vi "Current_Calib_Filenames.vi"(3 "Calib Filename":path[](array[path]), 4 "Channel Numbers":string[](array[string]), 5 "Mode":T1) -> (0 "Calib Filename Out":path[](array[path]), 1 "Channel Numbers Out":string[](array[string]))   [LabVIEW 2013]
uses:
  Controls/App_Global.ctl
  File/Setup_Filetype.ctl
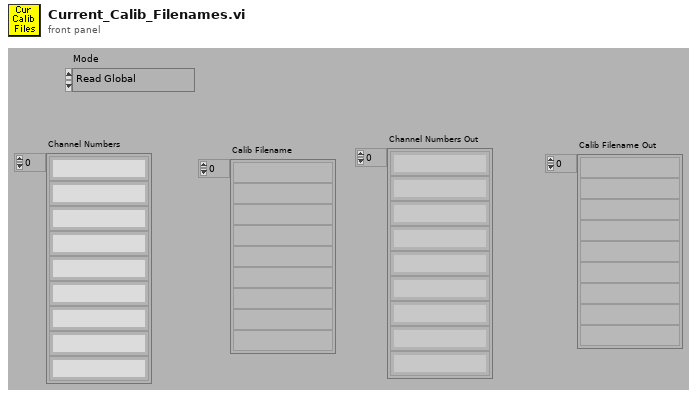
[diagram p1: front panel]
types:
  T1 = typedef "App_Global.ctl" = enum16{"Read Global", "Write to Global", "Initialise Array"}
  T2 = typedef "Setup_Filetype.ctl" = enum16{"Measurement Setups", "Calibration Setups", "General", "Results File Plotter Setups", "Speed Calib Tweaks"}
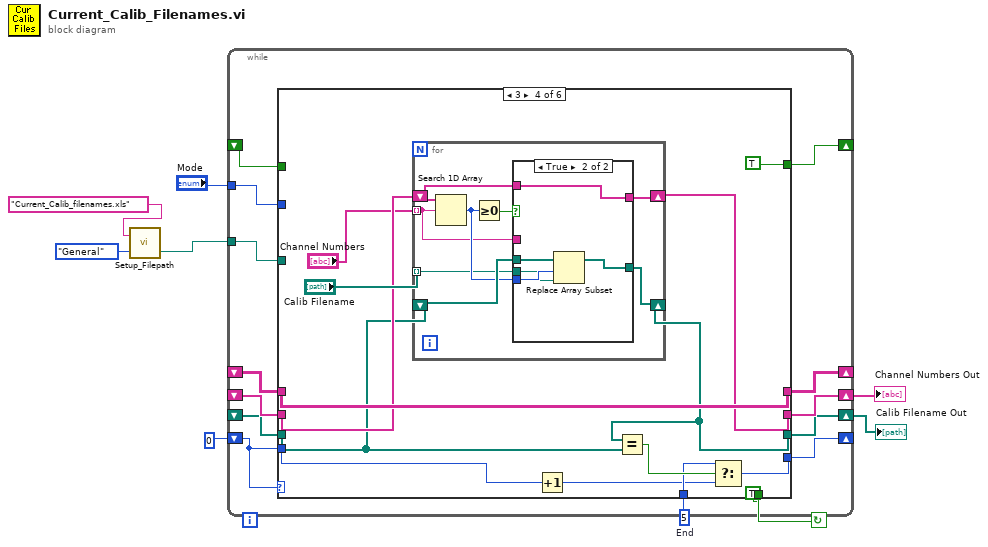
[diagram p0: block diagram]
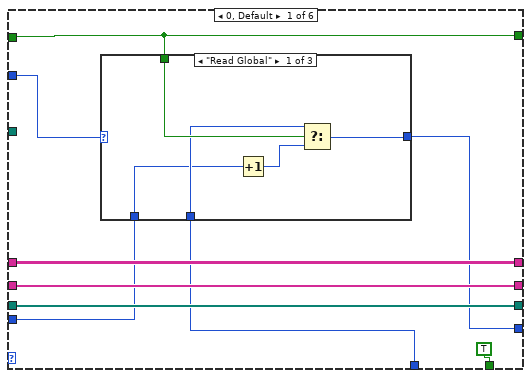
[diagram p2: hidden frame]
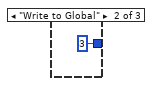
[diagram p3: hidden frame]
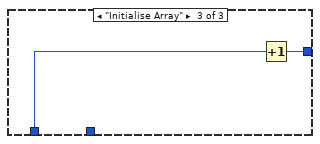
[diagram p4: hidden frame]
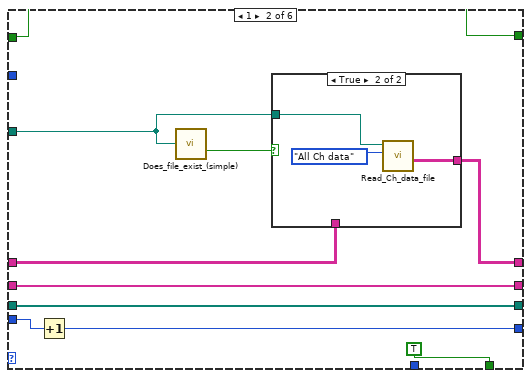
[diagram p5: hidden frame]
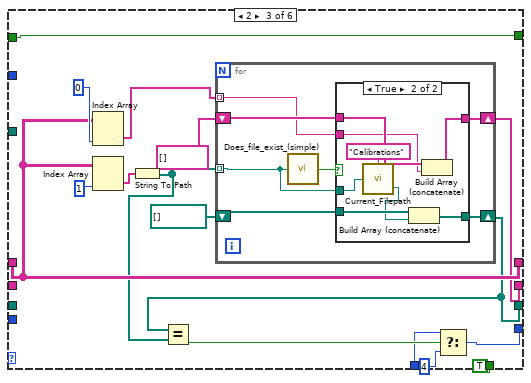
[diagram p7: hidden frame]
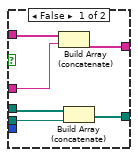
[diagram p9: hidden frame]
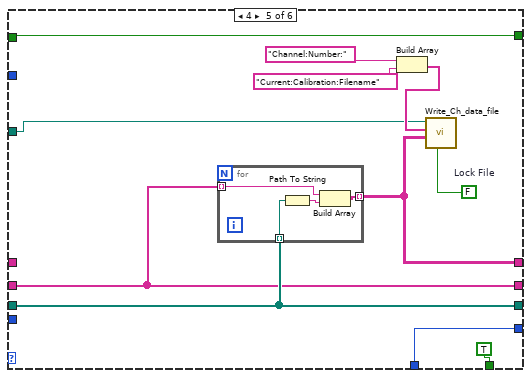
[diagram p10: hidden frame]
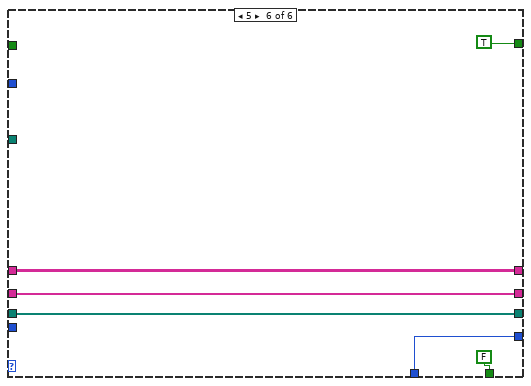
[diagram p11: hidden frame]
diagram:
  n1 = call "Setup_Filepath.vi"("Setup File Type"=Setup_Filetype."General", "Filename in"="Current_Calib_filenames.xls" ("Substring")) -> ("Filename Out"=w3:path)  [unwired: 1 out]
  n2 = while {
    shift-left: _ -> [w10]
    shift-right: [w12] -> w5
    shift-left: _ -> [w11]
    shift-right: [w13] -> w1
    tunnel: "Mode" -> [w17]
    shift-left: 0 -> [w18]
    shift-right: [w19] -> _
    shift-left: _ -> [w14]
    shift-right: [w15] -> _
    shift-left: _ -> [w21]
    shift-right: [w16] -> _
    tunnel: w3 -> [w8]
    stop <- w20 continue-if-true
    w9 = 5  # End
    n3 = case shown="3" w18 {
      tunnel: w21 -> [w25 w45 w64 _ w129 _]
      tunnel: [TRUE TRUE TRUE TRUE TRUE FALSE] -> w20
      tunnel: [w22 w46 w56 w87 w128 w135] -> w19
      tunnel: w18 -> [w23 w47 _ w89 _ _]
      tunnel: w17 -> [w26 _ _ _ _ _]
      tunnel: [w25 w45 w64 TRUE w129 TRUE] -> w16
      tunnel: [w28 w43 w63 w98 w121 w138] -> w15
      tunnel: w14 -> [w28 w42 w63 w98 _ w138]
      tunnel: [w30 w41 w61 w94 w122 w137] -> w13
      tunnel: [w29 w40 w60 w93 w123 w136] -> w12
      tunnel: w11 -> [w30 w41 _ w95 w122 w137]
      tunnel: w10 -> [w29 w40 _ w92 w123 w136]
      tunnel: w9 -> [w24 _ w57 w90 w128 w135]
      tunnel: w8 -> [_ w39 _ _ w119 _]
      frame 0, Default {
        n4 = case shown="\"Read Global\"" w26 {
          tunnel: w25 -> [w35 _ _]
          tunnel: w24 -> [w34 _ _]
          tunnel: w23 -> [w32 _ w38]
          tunnel: [w31 3 ("End") w37] -> w22
          frame "Read Global" {
            n5 = Increment(x=w32) -> (x+1=w33:i32)
            n6 = Select(t=w34, s=w35, f=w33) -> (s? t:f=w31:i32)
          }
          frame "Write to Global" {
          }
          frame "Initialise Array" {
            n7 = Increment(x=w38) -> (x+1=w37:i32)
          }
        }
      }
      frame 1 {
        n8 = Increment(x=w47) -> (x+1=w46:i32)
        n9 = call "Does_file_exist_(simple).vi"("Pathname"=w39) -> ("exists?"=w44:bool)
        n10 = case shown="True" w44 {
          tunnel: w39 -> [_ w51]
          tunnel: [w49 w50] -> w43
          tunnel: w42 -> [w49 _]
          frame False {
          }
          frame True {
            n11 = call "Read_Ch_data_file.vi"("Output"=enum16{"All Ch data", "The last few rows"}."All Ch data", "Filename"=w51) -> ("Channel Values"=w50:string[][])  [unwired: 3 in, 4 out]
          }
        }
      }
      frame 2 {
        n12 = Index Array(array=w63, index (col)=0 ("Index")) -> (element=w54:string[])  [unwired: 1 in]
        n13 = Index Array(array=w63, index (col)=1 ("Index")) -> (element=w65:string[])  [unwired: 1 in]
        n14 = String To Path(string=w65) -> (path=w59:path[])
        n15 = for {
          shift-right: [w73] -> w61
          shift-right: [w70] -> w60
          shift-left: path[] [] -> [w71]
          tunnel: w59 -> [w69] mode=indexing
          shift-left: string[] [] -> [w74]
          tunnel: w54 -> [w72] mode=indexing
          n16 = call "Does_file_exist_(simple).vi"("Pathname"=w69) -> ("exists?"=w75:bool)
          n17 = case shown="True" w75 {
            tunnel: w74 -> [w77 w85]
            tunnel: [w77 w84] -> w73
            tunnel: w72 -> [_ w78]
            tunnel: w71 -> [w76 w83]
            tunnel: [w76 w82] -> w70
            tunnel: w69 -> [_ w81]
            frame False {
            }
            frame True {
              n18 = call "Current_Filepath.vi"("Filename in"=w81, "Data Type"="Calibrations") -> ("Filename Out"=w79:path)  [unwired: 1 out]
              n19 = Build Array (concatenate)(w83, w79) -> (w82:path[])
              n20 = Build Array (concatenate)(w85, w78) -> (w84:string[])
            }
          }
        }
        n21 = Equal?(x=w60, y=w59) -> (x = y?=w58:bool)
        n22 = Select(t=w57, s=w58, f=4) -> (s? t:f=w56:i32)
      }
      frame 3 {
        n23 = for {
          tunnel: "Channel Numbers" -> [w100] mode=indexing
          shift-right: [w103] -> w93
          shift-left: w92 -> [w106]
          tunnel: "Calib Filename" -> [w104] mode=indexing
          shift-right: [w102] -> w94
          shift-left: w95 -> [w101]
          n24 = Search 1D Array(1D array=w101, element=w100) -> (index of element=w105:i32)  [unwired: 1 out]
          n25 = Greater Or Equal To 0?(x=w105) -> (x >= 0?=w107:bool)
          n26 = case shown="True" w107 {
            tunnel: w106 -> [w110 w118]
            tunnel: w105 -> [_ w117]
            tunnel: w104 -> [w109 w116]
            tunnel: [w108 w115] -> w103
            tunnel: [w111 w114] -> w102
            tunnel: w101 -> [w113 w114]
            tunnel: w100 -> [w112 _]
            frame False {
              n27 = Build Array (concatenate)(w113, w112) -> (w111:string[])
              n28 = Build Array (concatenate)(w110, w109) -> (w108:path[])
            }
            frame True {
              n29 = Replace Array Subset(array=w118, new element=w116, index=w117) -> (w115:path[])
            }
          }
        }
        n30 = Increment(x=w89) -> (x+1=w88:i32)
        n31 = Equal?(x=w93, y=w92) -> (x = y?=w91:bool)
        n32 = Select(t=w90, s=w91, f=w88) -> (s? t:f=w87:i32)
      }
      frame 4 {
        w120 = FALSE  # Lock File
        n33 = for {
          tunnel: w123 -> [w133] mode=indexing
          tunnel: w122 -> [w130] mode=indexing
          tunnel: [w132] -> w121 mode=indexing
          n34 = Path To String(path=w133) -> (string=w131:string)
          n35 = Build Array(w130, w131) -> (w132:string[])
        }
        n36 = Build Array("Channel:Number:", "Current:Calibration:Filename") -> (w124:string[])
        n37 = call "Write_Ch_data_file.vi"("Lock File"=w120, "Channel Values"=w121, "Channel names"=w124, "Filename"=w119) -> ()  [unwired: 4 in, 4 out]
      }
      frame 5 {
      }
    }
  }
  "Channel Numbers Out" <- w1
  "Calib Filename Out" <- w5
